vi "main.vi"() -> ()   [LabVIEW 2021]
uses:
  <vilib>/Waveform/WDTFileIO.llb/Export Waveforms To Spreadsheet File (1D).vi
panel:
  in  "Save File":bool
  out "Thermistor Unfiltered 2":waveform(dbl)[](graph)
  out "XY Graph":cluster{timestamp[], "Y":dbl[]}[](graph)
  out "Thermistor Filtered":T1(graph)
  out "Thermistor Unfiltered":T1(graph)
  in  "Thermistor":T2
  out "Waveform Chart 3":T3(graph)
  in  "error in (no error)":errorcluster
  out "error out":errorcluster
  out "Waveform Chart 2":waveform(dbl)(graph)
  out "a0 Scalar":dbl
  out "Waveform Chart":dynamicdata(graph)
  in  "stop":bool
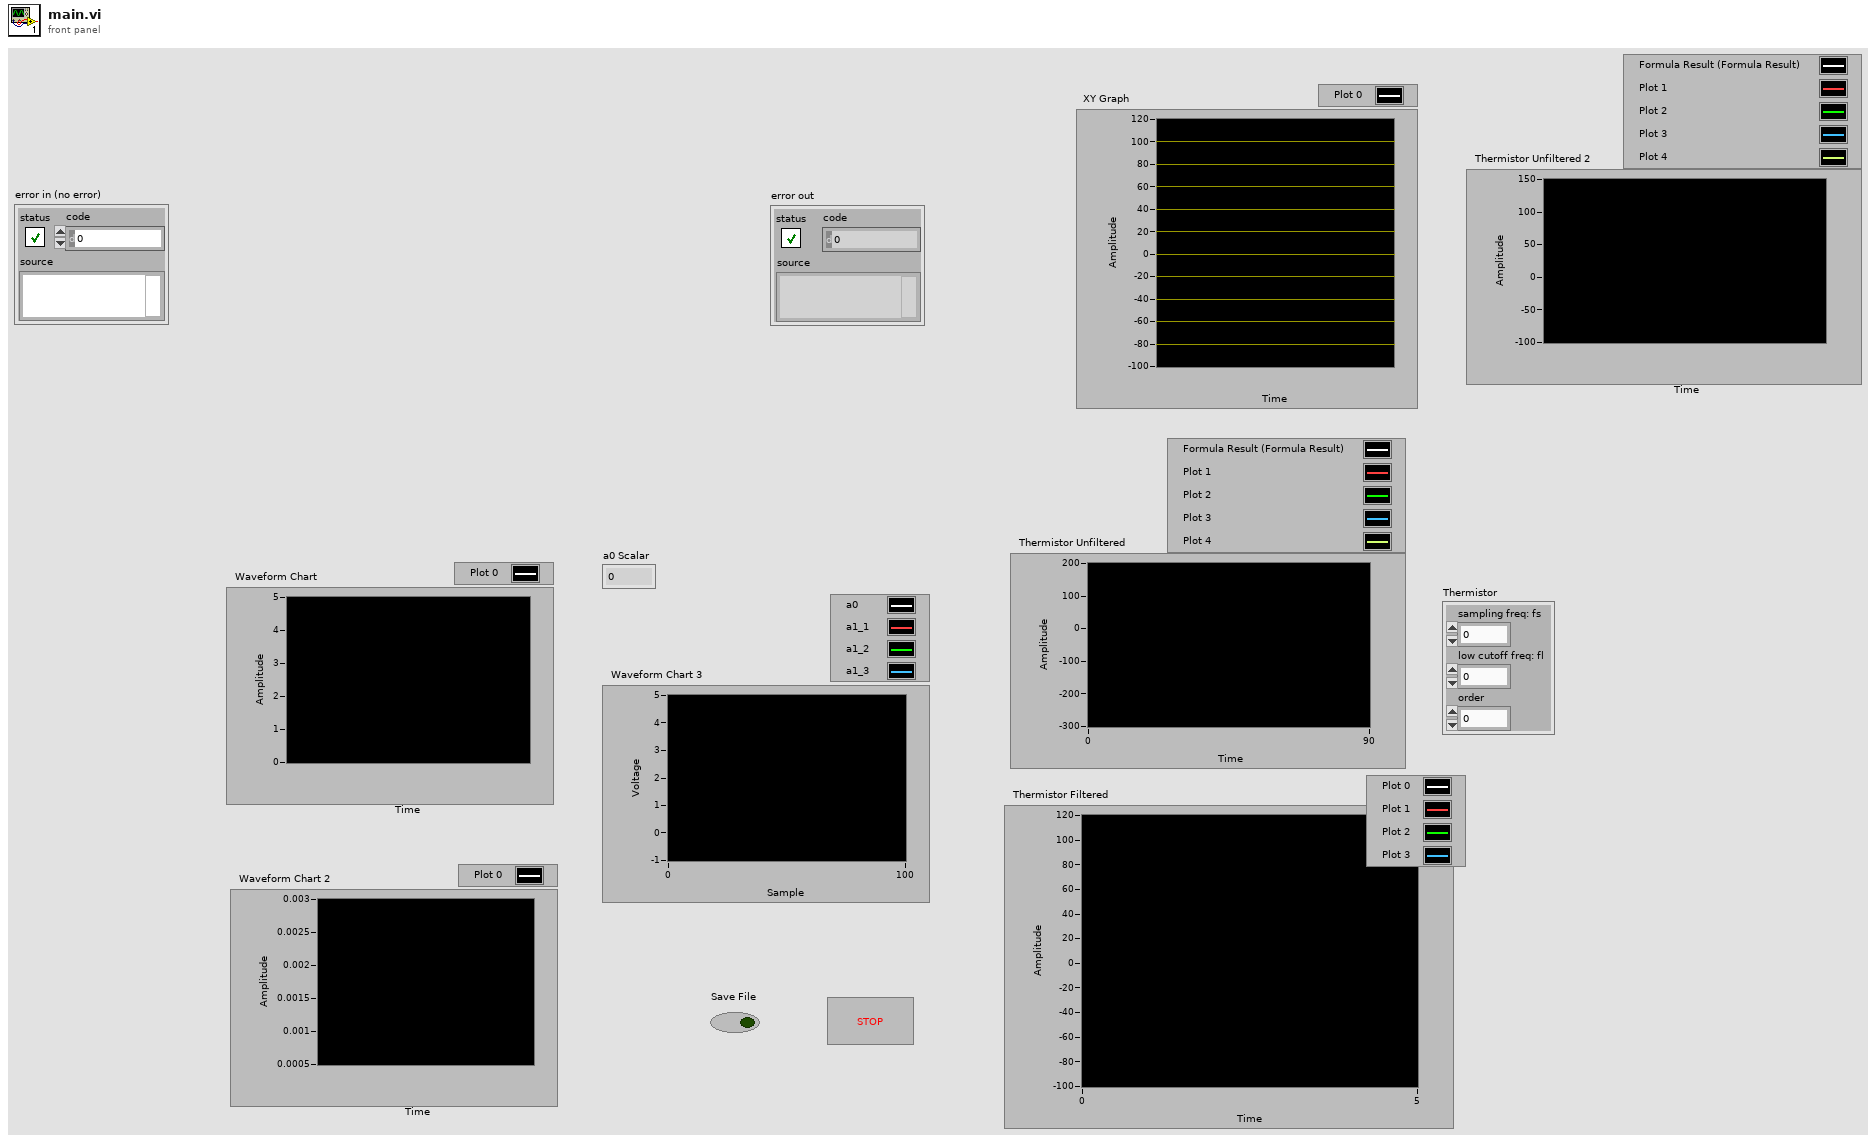
[diagram p1: front panel]
types:
  T1 = cluster{"[0]":dbl, "[1]":dbl, "[2]":dbl, "[3]":dbl, "[4]":dbl, "[5]":dbl, "[6]":dbl, "[7]":dbl, "[8]":dbl}
  T2 = cluster{"sampling freq: fs":dbl, "low cutoff freq: fl":dbl, "order":i32}
  T3 = cluster{"Data_Array[0]":dbl, "Data_Array[1]":dbl, "Data_Array[2]":dbl, "Data_Array[3]":dbl, "Data_Array[4]":dbl, "Data_Array[5]":dbl, "Data_Array[6]":dbl, "Data_Array[7]":dbl, "Data_Array[8]":dbl}
  T4 = cluster{"Data_Array":dbl[], "Multiplex_Tbl":u32[]}
  T5 = cluster{"Temp Filtered[0]":dbl, "Temp Filtered[1]":dbl, "Temp Filtered[2]":dbl, "Temp Filtered[3]":dbl, "Temp Filtered[4]":dbl, "Temp Filtered[5]":dbl, "Temp Filtered[6]":dbl, "Temp Filtered[7]":dbl, "Temp Filtered[8]":dbl}
  T6 = cluster{"Temp[0]":dbl, "Temp[1]":dbl, "Temp[2]":dbl, "Temp[3]":dbl, "Temp[4]":dbl, "Temp[5]":dbl, "Temp[6]":dbl, "Temp[7]":dbl, "Temp[8]":dbl}
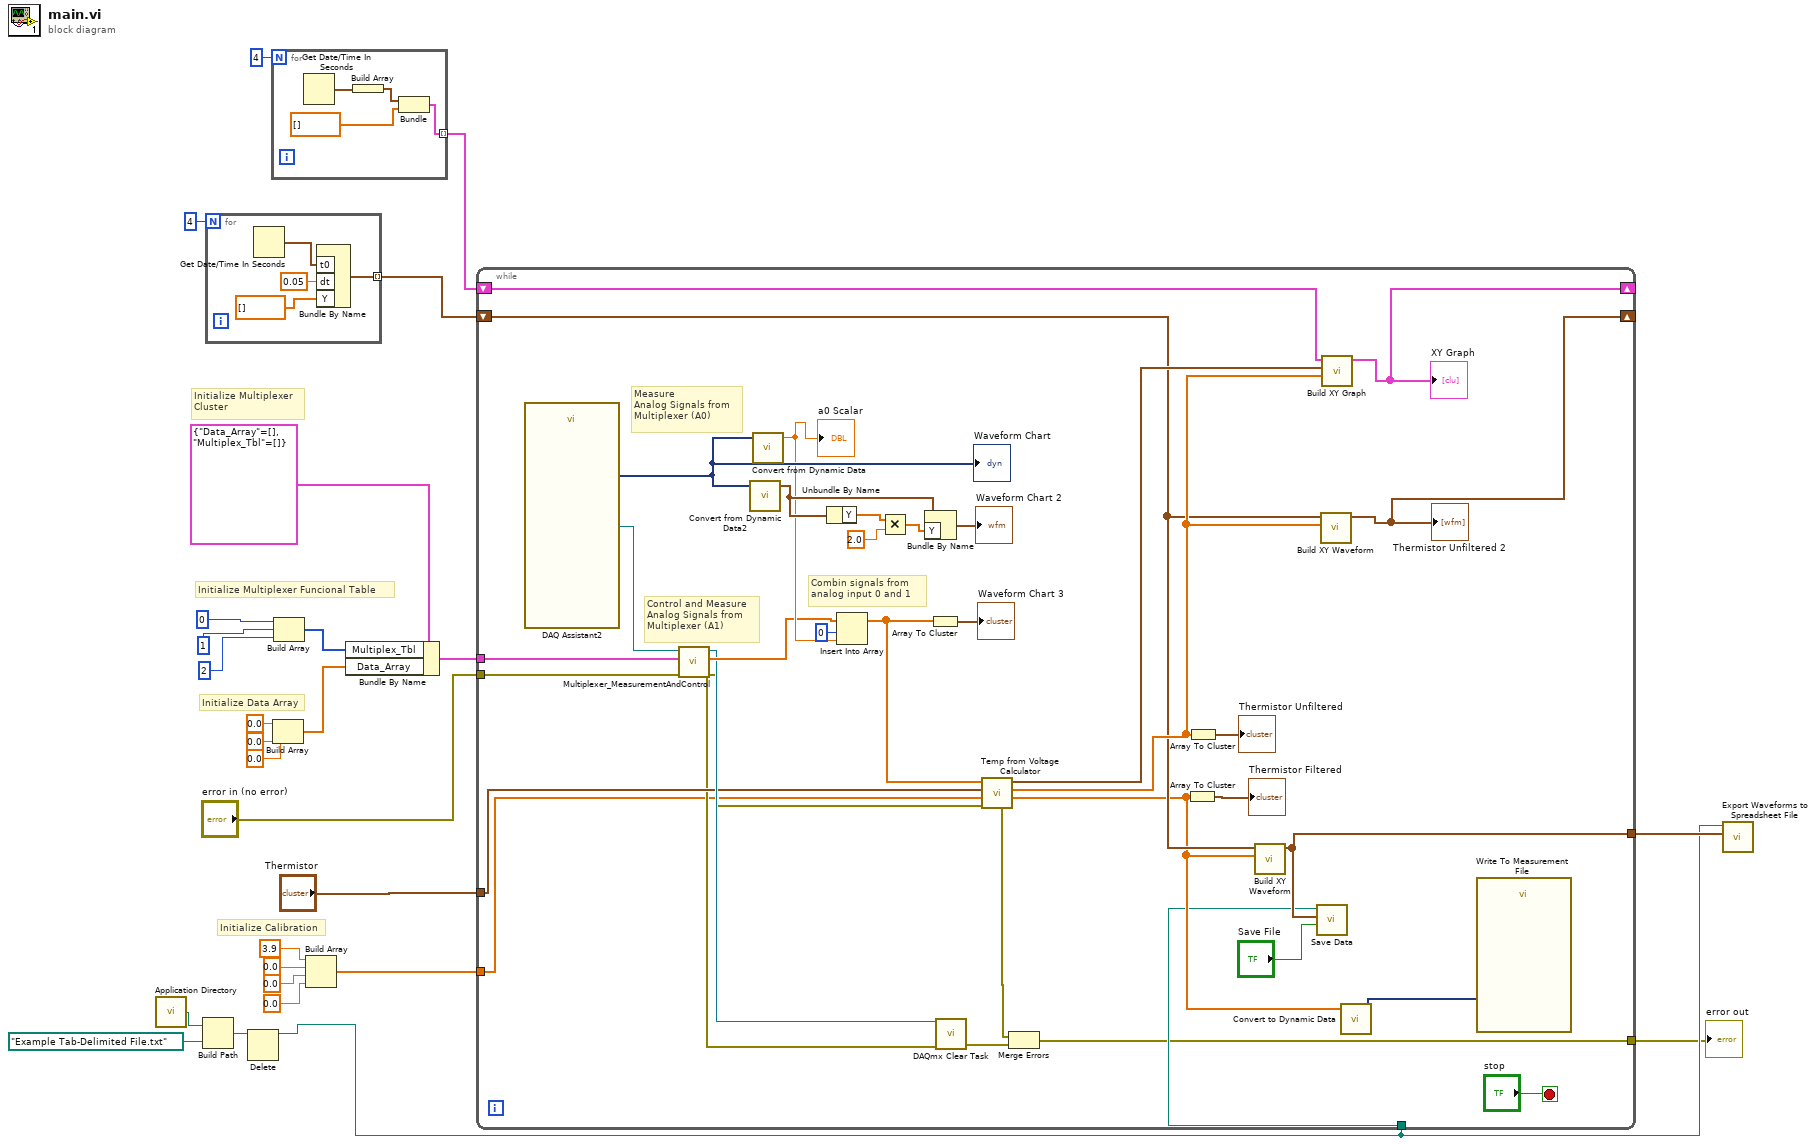
[diagram p0: block diagram]
diagram:
  # "Initialize Calibration"
  # "Initialize Multiplexer \nCluster"
  # "Initialize Data Array"
  # "Initialize Multiplexer Funcional Table"
  n1 = call <vilib>:"Application Directory.vi"() -> ("Application Directory"=w1:path)
  n2 = Build Path(base path=w1, name or relative path=path "Example Tab-Delimited File.txt" ("default name")) -> (appended path=w11:path)
  n3 = for {
    N: 4 -> [_]
    tunnel: [w28] -> w12 mode=indexing
    n4 = Get Date/Time In Seconds() -> (seconds since 1Jan1904=w30:timestamp)
    n5 = Bundle By Name("t0"=w30, "dt"=0.05, "Y"=dbl[] []) -> (w28:waveform(dbl))  [unwired: 1 in]
  }
  n6 = Delete(path (use dialog)=w11) -> (deleted path=w3:path)  [unwired: 4 in, 2 out]
  n7 = for {
    N: 4 -> [_]
    tunnel: [w33] -> w15 mode=indexing
    n8 = Get Date/Time In Seconds() -> (seconds since 1Jan1904=w35:timestamp)
    n9 = Build Array(w35) -> (w34:timestamp[])
    n10 = Bundle(w34, "Y"=dbl[] []) -> (w33:cluster{timestamp[], "Y":dbl[]})  [unwired: 1 in]
  }
  n11 = Build Array(0.0 ("element"), 0.0 ("element"), 0.0 ("element")) -> (w23:dbl[])
  n12 = Build Array(u32 0 ("Waveform"), 1 ("Waveform"), u32 2 ("Waveform")) -> (w17:u32[])
  n13 = Build Array(3.9 ("element"), 0.0 ("element"), 0.0 ("element"), 0.0 ("element")) -> (w4:dbl[])
  n14 = Bundle By Name(cluster=T4 {"Data_Array"=[], "Multiplex_Tbl"=[]}, "Multiplex_Tbl"=w17, "Data_Array"=w23) -> (w22:T4)
  n15 = while {
    tunnel: w22 -> [w63]
    tunnel: "error in (no error)" -> [w62]
    tunnel: "Thermistor" -> [w55]
    shift-right: [w49] -> _
    shift-left: w15 -> [w50]
    shift-right: [w47] -> _
    shift-left: w12 -> [w41]
    tunnel: [w38] -> w9
    tunnel: w4 -> [w42]
    tunnel: w3 -> [w37]
    tunnel: [w36] -> w2
    stop <- "stop" stop-if-true
    # "Combin signals from \nanalog input 0 and 1"
    # "Measure\nAnalog Signals from\nMultiplexer (A0)"
    # "Control and Measure\nAnalog Signals from\nMultiplexer (A1)"
    n16 = call "DAQ Assistant2"() -> ("task out"=w61:refnum<k21>, "data"=w64:dynamicdata)  [unwired: 16 in, 2 out]
    "Waveform Chart" <- w64
    n17 = call "Multiplexer_MeasurementAndControl.vi"("error in (no error)"=w62, "Multiplexer_Cluser"=w63, "Task in"=w61) -> ("error out"=w46:errorcluster, "Data_Array"=w58:dbl[], "Task out"=w56:refnum<k21>)  [unwired: 6 in]
    n18 = call "Convert from Dynamic Data2"("Dynamic Data Type"=w64) -> ("Waveform"=w67:waveform(dbl))  [unwired: 3 in]
    n19 = call "Convert from Dynamic Data"("Dynamic Data Type"=w64) -> ("Scalar"=w60:dbl)  [unwired: 3 in]
    "a0 Scalar" <- w60
    n20 = Unbundle By Name(w67) -> ("Y"=w69:dbl[])
    n21 = Insert Into Array(array=w58, index=0, new element=w60) -> (w54:dbl[])
    n22 = Multiply(x=w69, y=2.0) -> (x*y=w66:dbl[])
    n23 = Bundle By Name(cluster=w67, "Y"=w66) -> (→"Waveform Chart 2":waveform(dbl))
    n24 = Array To Cluster(array=w54) -> (cluster=→"Waveform Chart 3":T3)
    n25 = call <vilib>:"DAQmx Clear Task.vi"("task in"=w56, "error in"=w46) -> ("error out"=w45:errorcluster)  [unwired: 13 in]
    n26 = call "Temp from Voltage Calculator.vi"("error in (no error)"=w46, "Calibrations"=w42, "Thermistor"=w55, "Data_Array"=w54) -> ("Temp Filtered"=w40:dbl[], "Temp"=w48:dbl[], "Time Read"=w43:timestamp[], "error out"=w44:errorcluster[])  [unwired: 4 in]
    n27 = Merge Errors(w44, w45) -> (w36:errorcluster)
    n28 = Array To Cluster(array=w40) -> (cluster=→"Thermistor Filtered":T5)
    n29 = Array To Cluster(array=w48) -> (cluster=→"Thermistor Unfiltered":T6)
    n30 = call "Build XY Waveform.vi"("New Temps"=w40, "Waveforms in"=w41) -> ("Waveforms out"=w38:waveform(dbl)[])  [unwired: 9 in]
    n31 = call "Save Data.vi"("Save File"="Save File", "Waveforms in"=w38, "deleted path"=w37) -> ()  [unwired: 9 in]
    n32 = call "Build XY Waveform.vi"("New Temps"=w48, "Waveforms in"=w41) -> ("Waveforms out"=w47:waveform(dbl)[])  [unwired: 9 in]
    "Thermistor Unfiltered 2" <- w47
    n33 = call "Build XY Graph.vi"("Meas Temp"=w48, "Meas Time"=w43, "XY In"=w50) -> ("XY out"=w49:cluster{timestamp[], "Y":dbl[]}[])  [unwired: 8 in]
    "XY Graph" <- w49
    n34 = call "Convert to Dynamic Data"("Array"=w40) -> ("Dynamic Data Type"=w53:dynamicdata)  [unwired: 3 in]
    n35 = call "Write To Measurement File"("Signals"=w53) -> ()  [unwired: 16 in, 3 out]
  }
  "error out" <- w2
  n36 = call-poly <vilib>:"Export Waveforms to Spreadsheet File.vi"("waveforms"=w9, "file path (dialog if empty)"=w3) -> ()  [unwired: 8 in, 2 out]
